vi "loadTestsFromTestCase.vi"(8 "error in (no error)":errorcluster, 10 "TestCase":refnum<class "TestCase.lvclass">, 11 "TestLoader in":refnum<class "TestLoader.lvclass">) -> (0 "error out":errorcluster, 2 "TestSuite":refnum<class "TestSuite.lvclass">, 3 "TestLoader out":refnum<class "TestLoader.lvclass">)   [LabVIEW 2019, in "TestLoader.lvclass"]
uses:
  TestLoader.lvclass
  TestCase/TestCase.lvclass
  TestSuite/TestSuite.lvclass
panel:
  # "JKI VI Tester for LabVIEW\nhttp://jkisoft.com/vi-tester\nCopyright (C) 2007-2009, JKI <info@jkisoft.com>\nALL RIGHTS RESERVED"
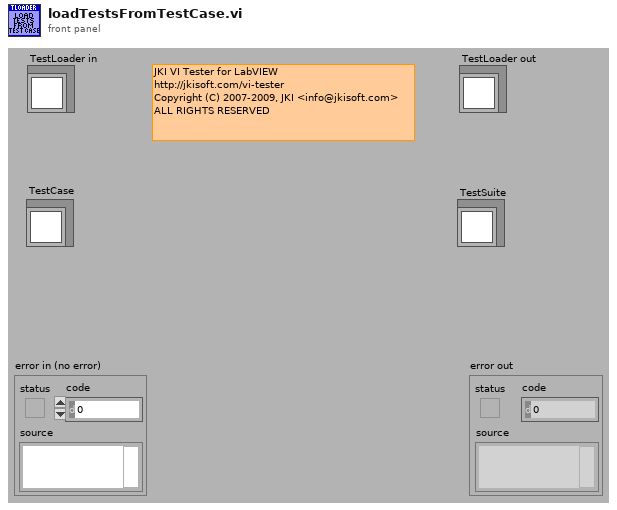
[diagram p1: front panel]
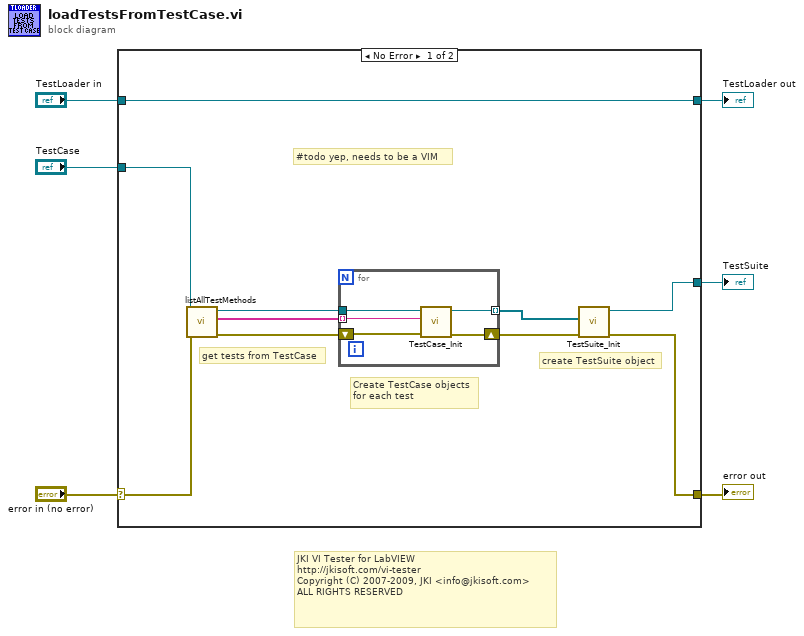
[diagram p0: block diagram]
diagram:
  # "JKI VI Tester for LabVIEW\nhttp://jkisoft.com/vi-tester\nCopyright (C) 2007-2009, JKI <info@jkisoft.com>\nALL RIGHTS RESERVED"
  n1 = case shown="No Error" "error in (no error)" {
    selector: "error in (no error)" -> [w10 w23]
    tunnel: [w12 w23] -> w5
    tunnel: [w16 w22] -> w3
    tunnel: "TestLoader in" -> [w16 w22]
    tunnel: "TestCase" -> [w11 _]
    tunnel: [w13 _] -> w1
    frame No Error {
      # "#todo yep, needs to be a VIM"
      # "create TestSuite object"
      # "Create TestCase objects\nfor each test"
      # "get tests from TestCase"
      n2 = call-dynamic "listAllTestMethods.vi"("error in (no error)"=w10, "TestCase in"=w11) -> ("error out"=w9:errorcluster, "test methods"=w8:string[], "TestCase out"=w7:refnum<class "TestCase.lvclass">)  [unwired: 7 in]
      n3 = for {
        tunnel: w7 -> [w21]
        tunnel: w8 -> [w20] mode=indexing
        shift-right: [w18] -> w15
        shift-left: w9 -> [w19]
        tunnel: [w17] -> w14 mode=indexing
        n4 = call "TestCase_Init.vi"("error in (no error)"=w19, "methodName (\"runTest\")"=w20, "TestCase in"=w21) -> ("error out"=w18:errorcluster, "TestCase out"=w17:refnum<class "TestCase.lvclass">)  [unwired: 7 in]
      }
      n5 = call "TestSuite_Init.vi"("error in (no error)"=w15, "tests (none)"=w14) -> ("error out"=w12:errorcluster, "TestSuite out"=w13:refnum<class "TestSuite.lvclass">)  [unwired: 8 in]
    }
    frame Error {
    }
  }
  "error out" <- w5
  "TestLoader out" <- w3
  "TestSuite" <- w1
